vi "WLAN - niVST - RFSA - Frequency and Level Settings.vi"(0 "instrument handle":refnum<k15>, 5 "TV Parameters(DataType)":T1 {"Tx_Chan" format="%.0x"; "Standard" items=["80211A/G/J/P OFDM", "80211B/G DSSS", "80211G DSSSOFDM", "80211N MIMOOFDM", "80211AC MIMOOFDM"]; "OFDM Data Rate (Mbps)" items=["6", "9", "12", "18", "24", "36", "48", "54"]; "80211n PLCP Frame Format" items=["Mixed Format", "Greenfield Format"]; "FEC Coding Type" items=["BCC", "LDPC"]; "DSSS Data Rate (Mbps)" items=["1", "2", "5.5 CCK", "5.5 PBCC", "11 CCK", "11 PBCC", "22", "33"]}, 7 "PL":dbl, 11 "error in":errorcluster) -> (4 "instrument handle":refnum<k15>, 15 "error out":errorcluster)   [LabVIEW 2011]
uses:
  TV/RW/Includes/WLAN - TV - RW - INC - TV_DataType_Cluster.ctl
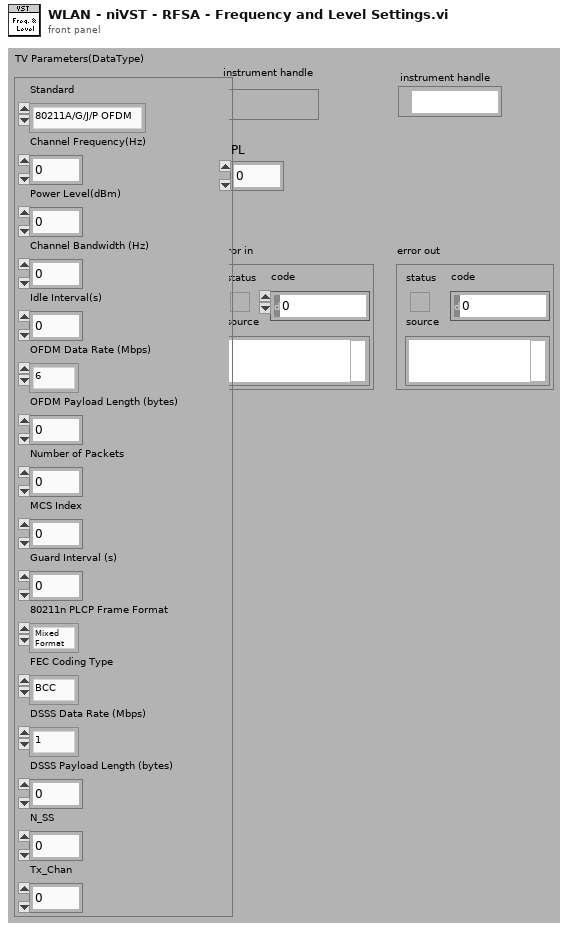
[diagram p1: front panel]
types:
  T1 = typedef "WLAN - TV - RW - INC - TV_DataType_Cluster.ctl" = cluster{"Standard":i32, "Channel Frequency(Hz)":dbl, "Power Level(dBm)":dbl, "Channel Bandwidth (Hz)":dbl, "Idle Interval(s)":dbl, "OFDM Data Rate (Mbps)":i32, "OFDM Payload Length (bytes)":i32, "Number of Packets":i32, "MCS Index":i32, "Guard Interval (s)":dbl, "80211n PLCP Frame Format":i32, "FEC Coding Type":i32, "DSSS Data Rate (Mbps)":i32, "DSSS Payload Length (bytes)":i32, "N_SS":i32, "Tx_Chan":u32}
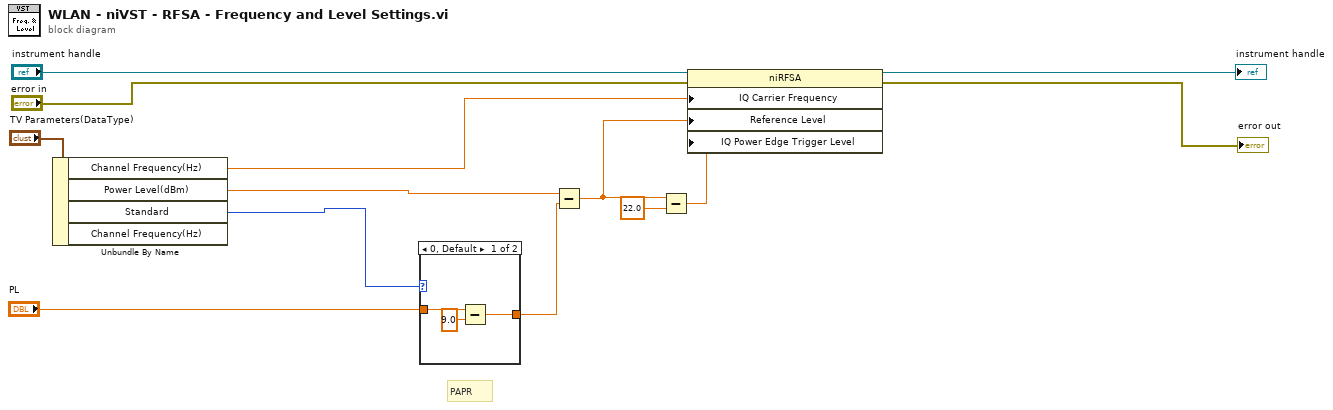
[diagram p0: block diagram]
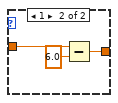
[diagram p2: hidden frame]
diagram:
  # "PAPR"
  n1 = Unbundle By Name("TV Parameters(DataType)") -> ("Channel Frequency(Hz)"=w6:dbl, "Power Level(dBm)"=w5:dbl, "Standard"=w3:i32)  [unwired: 1 out]
  n2 = case shown="0, Default" w3 {
    tunnel: "PL" -> [w16 w18]
    tunnel: [w14 w17] -> w2
    frame 0, Default {
      n3 = Subtract(x=w16, y=9.0) -> (x-y=w14:dbl)
    }
    frame 1 {
      n4 = Subtract(x=w18, y=6.0) -> (x-y=w17:dbl)
    }
  }
  n5 = Subtract(x=w5, y=w2) -> (x-y=w4:dbl)
  n6 = Subtract(x=w4, y=22.0) -> (x-y=w12:dbl)
  n7 = property class="niRFSA"(reference="instrument handle", error in="error in", "IQ Carrier Frequency"=w6, "Reference Level"=w4, "IQ Power Edge Trigger Level"=w12) -> (reference out=→"instrument handle":refnum<k15>, error out=→"error out":errorcluster)
